vi "Load Subitems.vi"(7 "defer fp updates?(T)":bool=TRUE, 8 "error in (no error)":errorcluster, 9 "Tag":string, 11 "Application Data in":T1) -> (0 "error out":errorcluster, 1 "item children":string[](array[string]), 3 "Application Data out":T1)   [LabVIEW 2020, in "DSF Configuration Utility.lvlib"]
uses:
  DSF Configuration Utility.lvlib
  ID to Tree Items/Tree Item Type.ctl
  Main VI/Application Data.ctl
  Main VI/View Mode.ctl
  Includes/DSF Core.lvlibp/Classes/Configuration Session/Configuration Session.lvclass
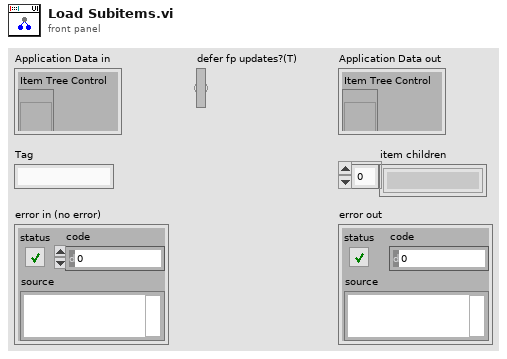
[diagram p1: front panel]
types:
  T1 = typedef "DSF Configuration Utility.lvlib/Application Data.ctl" = cluster{"Item Tree Control":refnum<vi>, "Value Tree Control":refnum<vi>, "Configuration Session":refnum<class "Configuration Session.lvclass">, "Top-Level VI":refnum<vi>, "View State":T2, "menu reference":refnum<k9>}
  T2 = typedef "DSF Configuration Utility.lvlib/View Mode.ctl" = enum16{"Tree", "List"}
  T3 = typedef "DSF Configuration Utility.lvlib/Tree Item Type.ctl" = enum16{"Plugin", "Group", "Transfer", "Channel", "Setting"}
  T4 = typedef "DSF Core.lvlibp/DSF Engine Plugin Configuration.ctl" = cluster{"name":string, "components":string[], "cycle timing":T5, "threads":T6[], "transfer groups":T8[], "settings":T7}
  T5 = typedef "DSF Core.lvlibp/DSF Timing Info.ctl" = cluster{"priority":u64, "decimation":u64, "offset":u64}
  T6 = typedef "DSF Core.lvlibp/DSF Engine Plugin Thread Configuration.ctl" = cluster{"processor":i32, "priority offset":i16, "settings":T7}
  T7 = typedef "DSF Core.lvlibp/DSF Settings Info.ctl" = cluster{"component":string, "name":string, "values":cluster{"key":string, "value":string}[]}[]
  T8 = typedef "DSF Core.lvlibp/DSF Engine Transfer Group Configuration.ctl" = cluster{"name":string, "direction":T9, "cycle timing":T5, "thread index":i32, "settings":T7, "transfers":T10[], "timeout behavior":T14}
  T9 = typedef "DSF Core.lvlibp/DSF Direction.ctl" = enum8{"Tx", "Rx"}
  T10 = typedef "DSF Core.lvlibp/DSF Engine Transfer Configuration.ctl" = cluster{"name":string, "byte order":T11, "settings":T7, "channels":T12[]}
  T11 = typedef "DSF Core.lvlibp/DSF Byte Order.ctl" = enum8{"big-endian", "little-endian"}
  T12 = typedef "DSF Core.lvlibp/DSF Engine Channel Configuration.ctl" = cluster{"string offset":u64, "name":string, "units":string, "engine data type":T13, "string data type":T13, "settings":T7}
  T13 = typedef "DSF Core.lvlibp/DSF Data Type.ctl" = enum8{"Bool", "SGL", "DBL", "I8", "I16", "I32", "I64", "U8", "U16", "U32", "U64"}
  T14 = typedef "DSF Core.lvlibp/DSF Timeout Behavior.ctl" = enum8{"Increment Late Count", "Throw Error"}
  T15 = typedef "DSF Configuration Utility.lvlib/Tree Item.ctl" = cluster{"Left Cell String":string, "Child Text":string[], "Child Tag":string, "Glyph Index":i32}
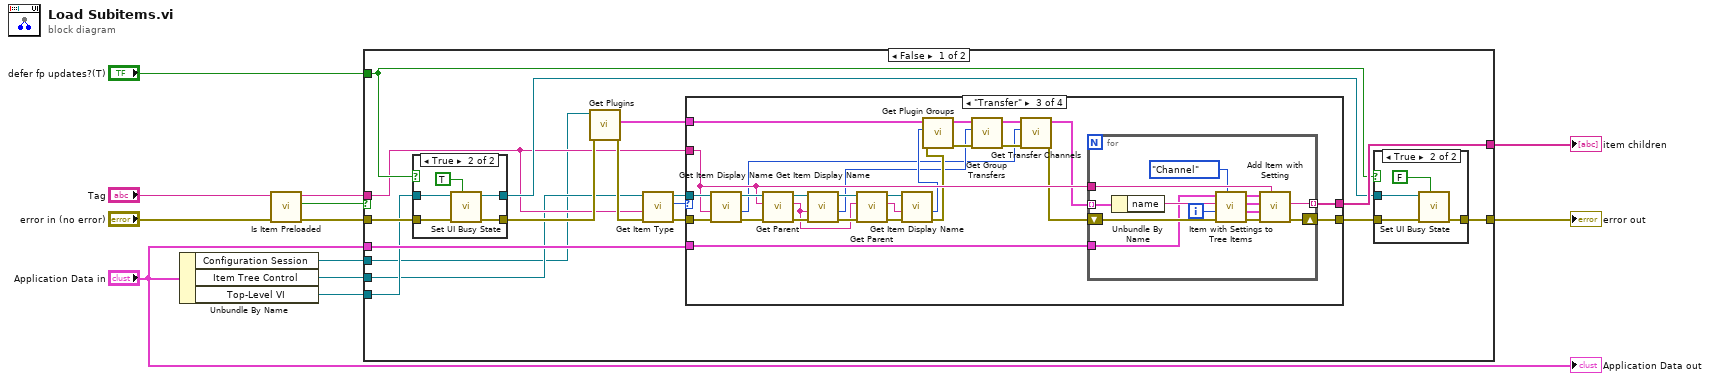
[diagram p0: block diagram]
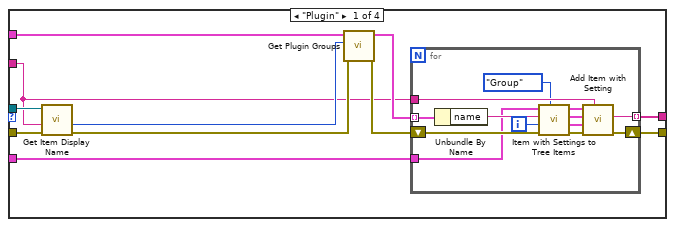
[diagram p4: hidden frame]
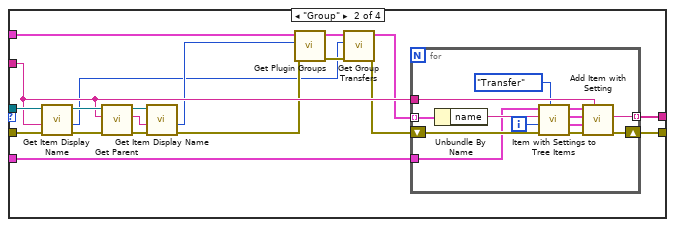
[diagram p5: hidden frame]
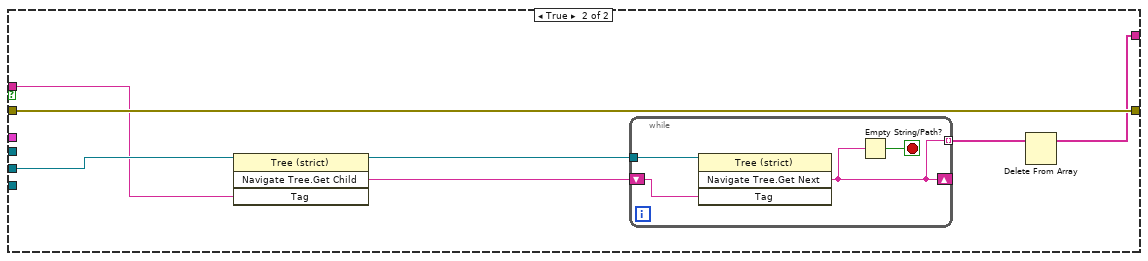
[diagram p7: hidden frame]
diagram:
  n1 = Unbundle By Name("Application Data in") -> ("Configuration Session"=w3:refnum<class "Configuration Session.lvclass">, "Item Tree Control"=w2:refnum<vi>, "Top-Level VI"=w1:refnum<vi>)
  n2 = call "Is Item Preloaded"("error in (no error)"="error in (no error)", "Tag in"="Tag") -> ("error out"=w4:errorcluster, "replaced"=w5:bool, "Tag out"=w6:string)  [unwired: 7 in]
  n3 = case shown="False" w5 {
    tunnel: w3 -> [w14 _]
    tunnel: w2 -> [w15 w143]
    tunnel: [w20 w144] -> w11
    tunnel: w4 -> [w24 w144]
    tunnel: w6 -> [w17 w142]
    tunnel: [w23 w139] -> w9
    tunnel: "Application Data in" -> [w21 _]
    tunnel: w1 -> [w16 _]
    tunnel: "defer fp updates?(T)" -> [w18 _]
    frame False {
      n4 = case shown="True" w18 {
        tunnel: w24 -> [w30 w35]
        tunnel: w16 -> [_ w34]
        tunnel: [w30 w33] -> w29
        tunnel: [_ w32] -> w19
        frame False {
        }
        frame True {
          n5 = call "Set UI Busy State.vi"("Defer Panel Updates"=TRUE, "error in (no error)"=w35, "VI in"=w34) -> ("error out"=w33:errorcluster, "VI out"=w32:refnum<vi>)  [unwired: 7 in]
        }
      }
      n6 = call "Get Plugins.vi"("error in (no error)"=w29, "configuration session in"=w14) -> ("error out"=w28:errorcluster, "plugins"=w13:T4[])  [unwired: 7 in, 1 out]
      n7 = call "Get Item Type.vi"("error in (no error)"=w28, "Tag"=w17, "TreeControl in"=w15) -> ("error out"=w27:errorcluster, "Item Type"=w26:T3, "TreeControl out"=w22:refnum<vi>)  [unwired: 6 in]
      n8 = case shown="\"Transfer\"" w26 {
        tunnel: w22 -> [w51 w83 w123 _]
        tunnel: w27 -> [w50 w82 w122 w137]
        tunnel: [w48 w80 w120 w137] -> w25
        tunnel: w17 -> [w41 w73 w113 _]
        tunnel: [w49 w81 w121 _] -> w23
        tunnel: w21 -> [w43 w78 w118 _]
        tunnel: w13 -> [w47 w79 w119 _]
        frame "Plugin" {
          n9 = call "Get Item Display Name.vi"("error in (no error)"=w50, "Tag"=w41, "TreeControl in"=w51) -> ("error out"=w45:errorcluster, "index"=w46:i32)  [unwired: 5 in, 2 out]
          n10 = call "Get Plugin Groups.vi"("error in (no error)"=w45, "plugin index"=w46, "plugins"=w47) -> ("error out"=w44:errorcluster, "transfer groups"=w42:T8[])  [unwired: 7 in]
          n11 = for {
            tunnel: w41 -> [w62]
            tunnel: [w63] -> w49 mode=indexing
            tunnel: w43 -> [w52]
            shift-right: [w64] -> w48
            shift-left: w44 -> [w59]
            tunnel: w42 -> [w54] mode=indexing
            i -> [w58]
            n12 = Unbundle By Name(w54) -> ("name"=w53:string)
            n13 = call "Item with Settings to Tree Items.vi"("item type"=Tree_Item_Type."Group", "error in (no error)"=w59, "item index"=w58, "item name"=w53, "Application Data in"=w52) -> ("error out"=w61:errorcluster, "Settings Item"=w57:T15, "Item"=w56:T15, "Application Data out"=w60:T1)  [unwired: 3 in]
            n14 = call "Add Item with Setting.vi"("Tag"=w62, "error in (no error)"=w61, "Setting"=w57, "Item"=w56, "Application Data in"=w60) -> ("error out"=w64:errorcluster, "new item tag"=w63:string)  [unwired: 4 in, 1 out]
          }
        }
        frame "Group" {
          n15 = call "Get Item Display Name.vi"("error in (no error)"=w82, "Tag"=w73, "TreeControl in"=w83) -> ("error out"=w75:errorcluster, "index"=w66:i32, "TreeControl out"=w74:refnum<vi>)  [unwired: 5 in, 1 out]
          n16 = call "Get Parent.vi"("error in (no error)"=w75, "tag"=w73, "TreeControl in"=w74) -> ("error out"=w71:errorcluster, "parent tag"=w70:string, "TreeControl out"=w72:refnum<vi>)  [unwired: 5 in, 1 out]
          n17 = call "Get Item Display Name.vi"("error in (no error)"=w71, "Tag"=w70, "TreeControl in"=w72) -> ("error out"=w68:errorcluster, "index"=w69:i32)  [unwired: 5 in, 2 out]
          n18 = call "Get Plugin Groups.vi"("error in (no error)"=w68, "plugin index"=w69, "plugins"=w79) -> ("error out"=w76:errorcluster, "transfer groups"=w77:T8[])  [unwired: 7 in]
          n19 = call "Get Group Transfers.vi"("error in (no error)"=w76, "group index"=w66, "transfer groups"=w77) -> ("error out"=w67:errorcluster, "transfers"=w65:T10[])  [unwired: 7 in]
          n20 = for {
            tunnel: w73 -> [w94]
            tunnel: [w95] -> w81 mode=indexing
            tunnel: w78 -> [w85]
            shift-right: [w96] -> w80
            shift-left: w67 -> [w91]
            tunnel: w65 -> [w84] mode=indexing
            i -> [w90]
            n21 = Unbundle By Name(w84) -> ("name"=w86:string)
            n22 = call "Item with Settings to Tree Items.vi"("item type"=Tree_Item_Type."Transfer", "error in (no error)"=w91, "item index"=w90, "item name"=w86, "Application Data in"=w85) -> ("error out"=w93:errorcluster, "Settings Item"=w89:T15, "Item"=w88:T15, "Application Data out"=w92:T1)  [unwired: 3 in]
            n23 = call "Add Item with Setting.vi"("Tag"=w94, "error in (no error)"=w93, "Setting"=w89, "Item"=w88, "Application Data in"=w92) -> ("error out"=w96:errorcluster, "new item tag"=w95:string)  [unwired: 4 in, 1 out]
          }
        }
        frame "Transfer" {
          n24 = call "Get Item Display Name.vi"("error in (no error)"=w122, "Tag"=w113, "TreeControl in"=w123) -> ("error out"=w115:errorcluster, "index"=w97:i32, "TreeControl out"=w114:refnum<vi>)  [unwired: 5 in, 1 out]
          n25 = call "Get Parent.vi"("error in (no error)"=w115, "tag"=w113, "TreeControl in"=w114) -> ("error out"=w111:errorcluster, "parent tag"=w106:string, "TreeControl out"=w112:refnum<vi>)  [unwired: 5 in, 1 out]
          n26 = call "Get Item Display Name.vi"("error in (no error)"=w111, "Tag"=w106, "TreeControl in"=w112) -> ("error out"=w108:errorcluster, "index"=w98:i32, "TreeControl out"=w107:refnum<vi>)  [unwired: 5 in, 1 out]
          n27 = call "Get Parent.vi"("error in (no error)"=w108, "tag"=w106, "TreeControl in"=w107) -> ("error out"=w109:errorcluster, "parent tag"=w110:string, "TreeControl out"=w105:refnum<vi>)  [unwired: 5 in, 1 out]
          n28 = call "Get Item Display Name.vi"("error in (no error)"=w109, "Tag"=w110, "TreeControl in"=w105) -> ("error out"=w99:errorcluster, "index"=w100:i32)  [unwired: 5 in, 2 out]
          n29 = call "Get Plugin Groups.vi"("error in (no error)"=w99, "plugin index"=w100, "plugins"=w119) -> ("error out"=w116:errorcluster, "transfer groups"=w117:T8[])  [unwired: 7 in]
          n30 = call "Get Group Transfers.vi"("error in (no error)"=w116, "group index"=w98, "transfer groups"=w117) -> ("error out"=w104:errorcluster, "transfers"=w102:T10[])  [unwired: 7 in]
          n31 = call "Get Transfer Channels.vi"("error in (no error)"=w104, "transfer index"=w97, "transfers"=w102) -> ("error out"=w103:errorcluster, "channels"=w101:T12[])  [unwired: 7 in]
          n32 = for {
            tunnel: w113 -> [w134]
            tunnel: [w135] -> w121 mode=indexing
            tunnel: w118 -> [w126]
            shift-right: [w136] -> w120
            shift-left: w103 -> [w131]
            tunnel: w101 -> [w125] mode=indexing
            i -> [w124]
            n33 = Unbundle By Name(w125) -> ("name"=w127:string)
            n34 = call "Item with Settings to Tree Items.vi"("item type"=Tree_Item_Type."Channel", "error in (no error)"=w131, "item index"=w124, "item name"=w127, "Application Data in"=w126) -> ("error out"=w133:errorcluster, "Settings Item"=w130:T15, "Item"=w129:T15, "Application Data out"=w132:T1)  [unwired: 3 in]
            n35 = call "Add Item with Setting.vi"("Tag"=w134, "error in (no error)"=w133, "Setting"=w130, "Item"=w129, "Application Data in"=w132) -> ("error out"=w136:errorcluster, "new item tag"=w135:string)  [unwired: 4 in, 1 out]
          }
        }
        frame "Channel", "Setting" {
        }
      }
      n36 = case shown="True" w18 {
        tunnel: w25 -> [w36 w40]
        tunnel: [w36 w39] -> w20
        tunnel: w19 -> [_ w38]
        frame False {
        }
        frame True {
          n37 = call "Set UI Busy State.vi"("Defer Panel Updates"=FALSE, "error in (no error)"=w40, "VI in"=w38) -> ("error out"=w39:errorcluster)  [unwired: 7 in, 1 out]
        }
      }
    }
    frame True {
      n38 = invoke class="Tree (strict)" method="Navigate Tree.Get Child"(reference=w143, "Tag"=w142) -> (reference out=w141:refnum<vi>, "Navigate Tree:Get Child"=w138:string)  [unwired: 2 in, 2 out]
      n39 = while {
        tunnel: w141 -> [w148]
        tunnel: [w145] -> w140 mode=indexing
        shift-right: [w145] -> _
        shift-left: w138 -> [w146]
        stop <- w147 stop-if-true
        n40 = invoke class="Tree (strict)" method="Navigate Tree.Get Next"(reference=w148, "Tag"=w146) -> ("Navigate Tree:Get Next Item"=w145:string)  [unwired: 2 in, 3 out]
        n41 = Empty String/Path?(string/path=w145) -> (empty?=w147:bool)
      }
      n42 = Delete From Array(array=w140) -> (array with subset deleted=w139:string[])  [unwired: 2 in, 1 out]
    }
  }
  "error out" <- w11
  "item children" <- w9
  "Application Data out" <- "Application Data in"
